vi "Searcher.vi"(7 "сегмент сигнала\nс SDR-приемника":cdb[](array[numeric])) -> (1 "CPICH convolution":dbl[](graph), 2 "PSC  convolution":dbl[](graph), 6 "l est":i32, 8 "I":cdb[](array[numeric]))   [LabVIEW 2017]
panel:
  out "p":i32
  in  "df steps":i32=2001
  # "df steps"
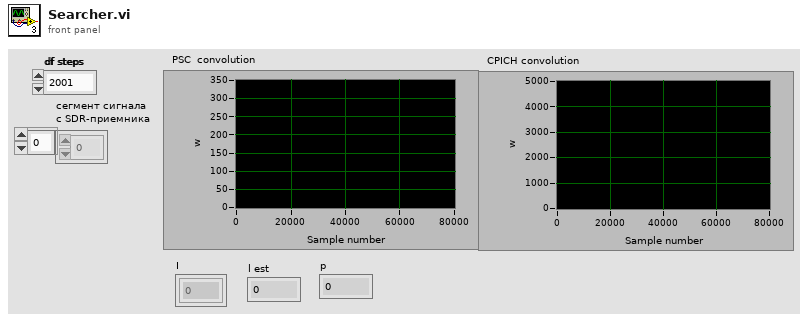
[diagram p1: front panel]
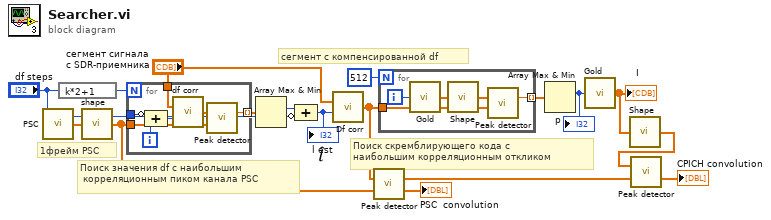
[diagram p0: block diagram]
diagram:
  # "Поиск скремблирующего кода с\nнаибольшим корреляционным откликом"
  # "1фрейм PSC"
  # "сегмент с компенсированной df"
  # "Поиск значения df с наибольшим \n корреляционным пиком канала PSC"
  n1 = call "PSC.vi"() -> ("Cpsc"=w9:cdb[])  [unwired: 15 in]
  n2 = expression code="k*2+1"("df steps") -> (w15:i32)
  n3 = call "shape.vi"("chips"=w9) -> ("envelope"=w5:cdb[])  [unwired: 14 in]
  n4 = for {
    N: w15 -> [_]
    tunnel: w5 -> [w19]
    tunnel: [w18] -> w16 mode=indexing
    tunnel: "df steps" -> [w23]
    tunnel: "сегмент сигнала\nс SDR-приемника" -> [w21]
    i -> [w22]
    n5 = Compound Arithmetic op=ADD(invert w23, w22) -> (w17:i32)
    n6 = call "df corr.vi"("in"=w21, "df"=w17) -> ("out"=w20:cdb[])  [unwired: 13 in]
    n7 = call "Peak detector.vi"("X"=w20, "Y"=w19) -> ("peak\nvalue"=w18:dbl)  [unwired: 11 in, 2 out]
  }
  n8 = Array Max & Min(array=w16) -> (max index (indices)=w11:i32)  [unwired: 3 out]
  n9 = Compound Arithmetic op=ADD(w11, invert "df steps") -> (w8:i32)
  "l est" <- w8
  n10 = call "Df corr.vi"("in"="сегмент сигнала\nс SDR-приемника", "df"=w8) -> ("out"=w2:cdb[])  [unwired: 13 in]
  n11 = call "Peak detector.vi"("X"=w2, "Y"=w5) -> ("r"=→"PSC  convolution":dbl[])  [unwired: 11 in, 2 out]
  n12 = for {
    N: 512 -> [_]
    tunnel: w2 -> [w25]
    tunnel: [w27] -> w13 mode=indexing
    i -> [w24]
    n13 = call "Gold.vi"("p"=w24) -> ("I"=w28:cdb[])  [unwired: 14 in]
    n14 = call "Shape.vi"("chips"=w28) -> ("envelope"=w26:cdb[])  [unwired: 14 in]
    n15 = call "Peak detector.vi"("X"=w26, "Y"=w25) -> ("peak\nvalue"=w27:dbl)  [unwired: 11 in, 2 out]
  }
  n16 = Array Max & Min(array=w13) -> (max index (indices)=w7:i32)  [unwired: 3 out]
  "p" <- w7
  n17 = call "Gold.vi"("p"=w7) -> ("I"=w3:cdb[])  [unwired: 14 in]
  "I" <- w3
  n18 = call "Shape.vi"("chips"=w3) -> ("envelope"=w1:cdb[])  [unwired: 14 in]
  n19 = call "Peak detector.vi"("X"=w1, "Y"=w2) -> ("r"=→"CPICH convolution":dbl[])  [unwired: 11 in, 2 out]
